vi "Initialize.vi"(7 "Serial Configuration":T1={"Baud Rate"=9600, "Parity"=0, "Data Bits"=8, "Stop Bits"=10, "Flow Control"=0} {"Flow Control" items=["None", "XON/XOFF", "RTS/CTS", "XON/XOFF & RTS/CTS", "DTR/DSR", "XON/XOFF & DTR/DSR"]; "Stop Bits" items=["1.0"=10, "1.5"=15, "2.0"=20]; "Data Bits" items=["7"=7, "8"=8]; "Parity" items=["None", "Odd", "Even", "Mark", "Space"]; "Baud Rate" items=["300"=300, "600"=600, "1200"=1200, "2400"=2400, "4800"=4800, "9600"=9600, "19200"=19200]}, 8 "error in (no error)":errorcluster, 9 "Reset (True)":bool=TRUE, 10 "ID Query (True)":bool=TRUE, 11 "VISA resource name":refnum<visa-resource-name>) -> (0 "error out":errorcluster, 3 "VISA resource name out":refnum<visa-resource-name>)   [LabVIEW 2020, in "Keithley 2600 Series.lvlib"]
doc: "Establishes communication with the instrument and optionally performs an instrument identification query and/or an instrument reset. It also places the instrument in a default state needed for other instrument driver operations. Therefore, call this VI before calling other instrument driver VIs for this instrument. Generally, you need to call the <b>Initialize</b> VI only once at the beginning of an application."
uses:
  Keithley 2600 Series.lvlib
panel:
  # "(c) 2020 National Instruments.  ALL RIGHTS RESERVED."
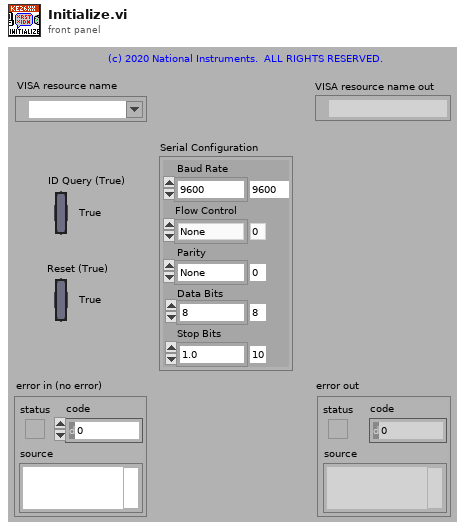
[diagram p1: front panel]
types:
  T1 = cluster{"Baud Rate":u32, "Parity":u16, "Data Bits":u16, "Stop Bits":u16, "Flow Control":u16}
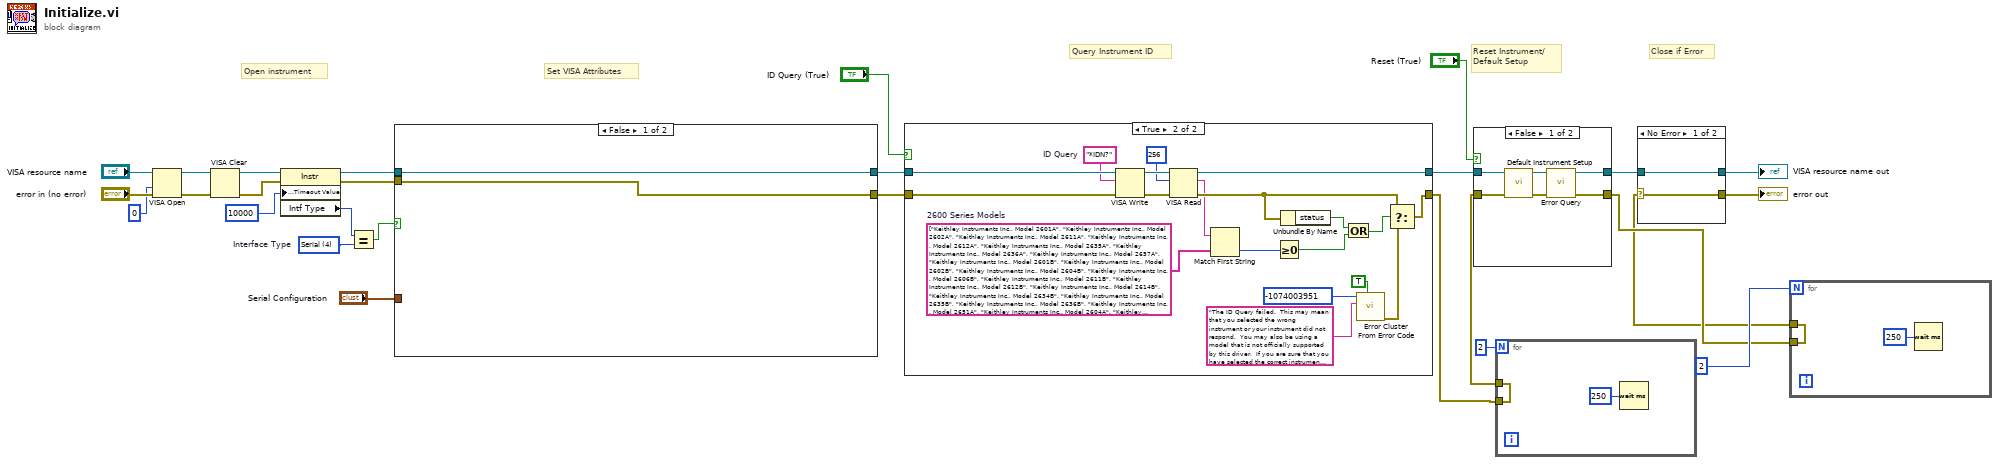
[diagram p0: block diagram]
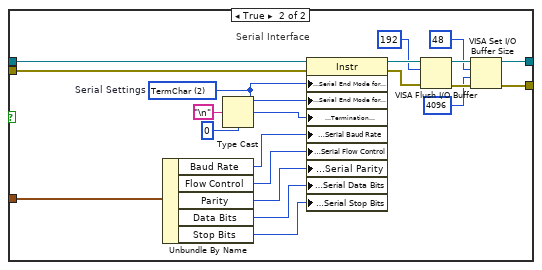
[diagram p2: hidden frame]
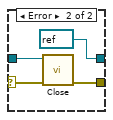
[diagram p3: hidden frame]
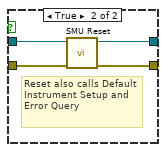
[diagram p4: hidden frame]
diagram:
  w14 = u16 4 items=["GPIB"=1, "VXI"=2, "GPIB-VXI"=3, "Serial"=4, "PXI"=5, "TCPIP"=6, "USB"=7]  # Interface Type
  # "Set VISA Attributes"
  # "Close if Error"
  # "Query Instrument ID"
  # "Reset Instrument/\nDefault Setup"
  # "Open instrument"
  n1 = VISA Open(access mode=u32 0, error in (no error)="error in (no error)", VISA resource name="VISA resource name") -> (VISA resource name=w21:refnum<visa-resource-name>, error out=w20:errorcluster)  [unwired: 2 in]
  n2 = VISA Clear(VISA resource name=w21, error in (no error)=w20) -> (VISA resource name out=w19:refnum<visa-resource-name>, error out=w18:errorcluster)
  n3 = property class="Instr"(reference=w19, error in=w18, "General Settings:Timeout Value"=u32 10000) -> (reference out=w12:refnum<visa-resource-name>, error out=w11:errorcluster, "Intf Type"=w13:u16)
  n4 = Equal?(x=w13, y=w14) -> (x = y?=w8:bool)
  n5 = case shown="False" w8 {
    tunnel: [w29 w48] -> w10
    tunnel: [w30 w45] -> w9
    tunnel: w12 -> [w29 w50]
    tunnel: w11 -> [w30 w51]
    tunnel: "Serial Configuration" -> [_ w31]
    frame False {
    }
    frame True {
      w38 = u16 2 items=["None", "LastBit", "TermChar"]  # Serial Settings
      # "Serial Interface"
      n6 = Unbundle By Name(w31) -> ("Baud Rate"=w36:u32, "Flow Control"=w33:u16, "Parity"=w34:u16, "Data Bits"=w35:u16, "Stop Bits"=w32:u16)
      n7 = Type Cast(type=u8 0, x="\n" ("Line Feed Constant")) -> (*(type *) &x=w37:u8)
      n8 = property class="Instr"(reference=w50, error in=w51, "Serial Settings:Serial End Mode for Reads"=w38, "Serial Settings:Serial End Mode for Writes"=w38, "Message Based Settings:Termination Character"=w37, "Serial Settings:Serial Baud Rate"=w36, "Serial Settings:Serial Flow Control"=w33, "Serial Settings:Serial Parity"=w34, "Serial Settings:Serial Data Bits"=w35, "Serial Settings:Serial Stop Bits"=w32) -> (reference out=w44:refnum<visa-resource-name>, error out=w47:errorcluster)
      n9 = VISA Flush I/O Buffer(VISA resource name=w44, mask (16)=u16 192, error in (no error)=w47) -> (VISA resource name out=w49:refnum<visa-resource-name>, error out=w46:errorcluster)
      n10 = VISA Set I/O Buffer Size(VISA resource name=w49, mask (16)=u16 48, size (4096)=u32 4096 ("size (0)"), error in (no error)=w46) -> (VISA resource name out=w48:refnum<visa-resource-name>, error out=w45:errorcluster)
    }
  }
  n11 = case shown="True" "ID Query (True)" {
    tunnel: [w52 w72] -> w5
    tunnel: [w53 w69] -> w28
    tunnel: w10 -> [w53 w70]
    tunnel: w9 -> [w52 w71]
    frame False {
    }
    frame True {
      w55 = string[] ["Keithley Instruments Inc., Model 2601A", "Keithley Instruments Inc., Model 2602A", "Keithley Instruments Inc., Model 2611A", "Keithley Instruments Inc., Model 2612A", "Keithley Instruments Inc., Model 2635A", "Keithley Instruments Inc., Model 2636A", "Keithley Instruments Inc., Model 2657A", "Keithley Instruments Inc., Model 2601B", "Keithley Instruments Inc., Model 2602B", "Keithley Instruments Inc., Model 2604B", "Keithley Instruments Inc., Model 2606B", "Keithley Instruments Inc., Model 2611B", "Keithley Instruments Inc., Model 2612B", "Keithley Instruments Inc., Model 2614B", "Keithley Instruments Inc., Model 2634B", "Keithley Instruments Inc., Model 2635B", "Keithley Instruments Inc., Model 2636B", "Keithley Instruments Inc., Model 2651A", "Keithley Instruments Inc., Model 2604A", "Keithley Instruments Inc., Model 2614A", "Keithley Instruments Inc., Model 2634A", "Keithley Instruments, Model 2601B-PULSE"]  # 2600 Series Models
      w65 = "*IDN?"  # ID Query
      n12 = VISA Write(VISA resource name=w70, write buffer=w65, error in (no error)=w71) -> (VISA resource name out=w68:refnum<visa-resource-name>, error out=w67:errorcluster)  [unwired: 1 out]
      n13 = VISA Read(VISA resource name=w68, byte count=u32 256, error in (no error)=w67) -> (VISA resource name out=w69:refnum<visa-resource-name>, read buffer=w54:string, error out=w60:errorcluster)  [unwired: 1 out]
      n14 = Match First String(2:w55, 3:w54) -> (0:w56:i32)  [unwired: 1 out]
      n15 = Greater Or Equal To 0?(x=w56) -> (x >= 0?=w58:bool)
      n16 = Unbundle By Name(w60) -> ("status"=w59:bool)
      n17 = Or(x=w59, y=w58) -> (x .or. y?=w57:bool)
      n18 = call <vilib>:"Error Cluster From Error Code.vi"("show call chain? (False)"=TRUE, "error message (\"\")"="The ID Query failed.  This may mean that you selected the wrong instrument or your instrument did not respond.  You may also be using a model that is not officially supported by this driver.  If you are sure that you have selected the correct instrument and it is responding, try disabling the ID Query." ("Source (VI Name)"), "error code (0)"=-1074003951 ("Code")) -> ("error out"=w64:errorcluster)  [unwired: 6 in]
      n19 = Select(t=w60, s=w57, f=w64) -> (s? t:f=w72:errorcluster)
    }
  }
  n20 = for {
    N: 2 -> [_]
    tunnel: w5 -> [w73]
    tunnel: [w73] -> w4
    n21 = Wait (ms)(milliseconds to wait=u32 250) -> ()  [unwired: 1 out]
  }
  n22 = case shown="False" "Reset (True)" {
    tunnel: w4 -> [w79 w82]
    tunnel: [w76 w81] -> w2
    tunnel: w28 -> [w80 w84]
    tunnel: [w77 w83] -> w15
    frame False {
      n23 = call "Default Instrument Setup.vi"("error in (no error)"=w79, "VISA resource name"=w80) -> ("error out"=w75:errorcluster, "VISA resource name out"=w78:refnum<visa-resource-name>)  [unwired: 8 in]
      n24 = call "Error Query.vi"("error in (no error)"=w75, "VISA resource name"=w78) -> ("error out"=w76:errorcluster, "VISA resource name out"=w77:refnum<visa-resource-name>)  [unwired: 6 in, 2 out]
    }
    frame True {
      # "Reset also calls Default Instrument Setup and Error Query"
      n25 = call "SMU Reset.vi"("error in (no error)"=w82, "VISA resource name"=w84) -> ("error out"=w81:errorcluster, "VISA resource name out"=w83:refnum<visa-resource-name>)  [unwired: 8 in]
    }
  }
  n26 = for {
    N: 2 -> [_]
    tunnel: w2 -> [w85]
    tunnel: [w85] -> w1
    n27 = Wait (ms)(milliseconds to wait=u32 250) -> ()  [unwired: 1 out]
  }
  n28 = case shown="No Error" w1 {
    selector: w1 -> [w87 w90]
    tunnel: w15 -> [w88 w91]
    tunnel: [w88 refnum<visa-resource-name> refnum ("VISA resource name out")] -> w17
    tunnel: [w87 w92] -> w16
    frame No Error {
    }
    frame Error {
      n29 = call "Close.vi"("error in (no error)"=w90, "VISA resource name"=w91) -> ("error out"=w92:errorcluster)  [unwired: 9 in]
    }
  }
  "VISA resource name out" <- w17
  "error out" <- w16
